vi "Get Graph Bounds.vi"(0 "eye scan point iterator":refnum<class "niHighSpeedSerial Rectangular Eye Scan Point Iterator v1 Host.lvclass">, 11 "error in":errorcluster) -> (4 "eye scan point iterator out":refnum<class "niHighSpeedSerial Rectangular Eye Scan Point Iterator v1 Host.lvclass">, 6 "x scale.range":T2, 8 "x scale.offset and multiplier":T1, 10 "y scale.range":T2, 14 "y scale.offset and multiplier":T1, 15 "error out":errorcluster)   [LabVIEW 2014, in "niHighSpeedSerial Rectangular Eye Scan Point Iterator v1 Host.lvclass"]
doc: "Returns the x, y, and z bounds to format an Intensity Graph based on the configuration of the Eye Scan Point Iterator object.\n\n<B>Input Parameters</B>\n\n<B>eye scan point iterator</B> is the incoming wire for the Eye Scan Point Iterator class object.\n\n<B>error in</B> describes error conditions that occur before this node runs. This input provides standard 'error in' functionality.\n\n<B>Output Parameters</B>\n\n<B>eye scan point iterator out</B> is the outgoing wire for the Eye Scan Point Iterator class object.\n\n<B>x scale.range</B> is the range for the x scale.\n\n<B>x scale.range.Minimum</B> is the minimum value for the x scale's range.\n\n<B>x scale.range.Maximum</B> is the maximum value for the x scale's range.\n\n<B>x scale.range.Increment</B> is the increment for the x scale's range.\n\n<B>x scale.range.Minor Increment</B> is the minor increment value for the x scale's range.\n\n<B>x scale.range.Start</B> is the start value for the x scale's range\n\n<B>x scale.offset and multiplier</B> is the offset and multiplier for the x scale's range.\n\n<B>x scale.offset and multiplier.Offset</B> is the offset for the x scale's range.\n\n<B>x scale.offset and multiplier.Multiplier</B> is the multiplier for the x scale's range.\n\n<B>y scale.range</B> is the range for the y scale.\n\n<B>y scale.range.Minimum</B> is the minimum value for the y scale's range.\n\n<B>y scale.range.Maximum</B> is the maximum value for the y scale's range.\n\n<B>y scale.range.Increment</B> is the increment for the y scale's range.\n\n<B>y scale.range.Minor Increment</B> is the minor increment for the y scale's range.\n\n<B>y scale.range.Start</B> is the start value for the y scale's range.\n\n<B>y scale.offset and multiplier</B> is the offset and multiplier for the y scale's range.\n\n<B>y scale.offset and multiplier.Offset</B> is the offset for the y scale's range.\n\n<B>y scale.offset and multiplier.Multiplier</B> is the multiplier for the y scale's range.\n\n<B>error out</B> contains error information. This output provides standard 'error out' functionality."
uses:
  <instrlib>/niHighSpeedSerial/Eye Scan/v1/Host/Impl/Rect Iter/niHighSpeedSerial Rectangular Eye Scan Point Iterator v1 Host.lvclass
  <vilib>/Utility/miscctls.llb/LVRangeTypeDef.ctl
  <vilib>/Utility/miscctls.llb/LVOffsetAndMultiplierTypeDef.ctl
  <instrlib>/niHighSpeedSerial/Eye Scan/v1/Host/Impl/Rect Iter/niHighSpeedSerial Rectangular Eye Scan Point Iterator v1 Host.lvclass/niHighSpeedSerial Rectangular Eye Scan Point Iterator v1 Host.ctl
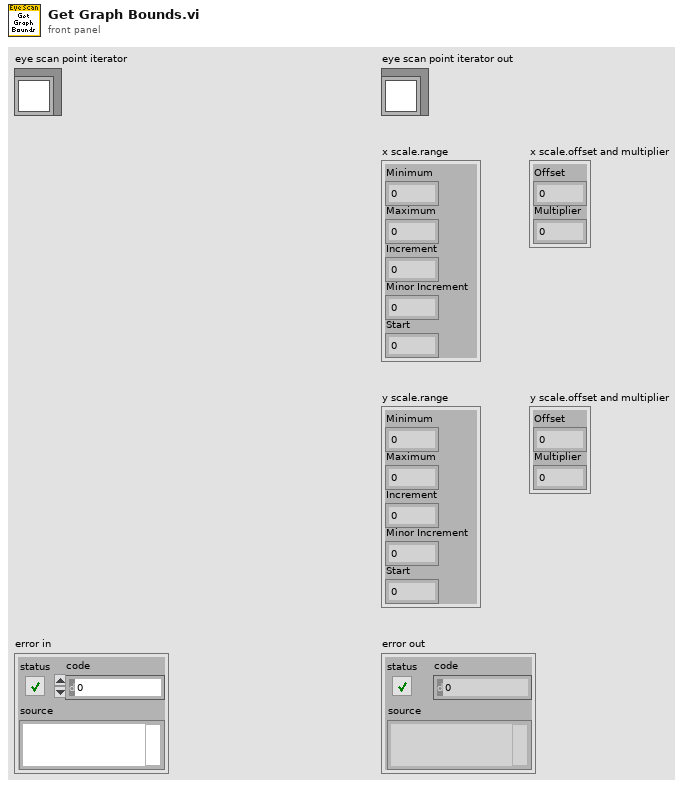
[diagram p1: front panel]
types:
  T1 = typedef "LVOffsetAndMultiplierTypeDef.ctl" = cluster{"Offset":dbl, "Multiplier":dbl}
  T2 = typedef "LVRangeTypeDef.ctl" = cluster{"Minimum":dbl, "Maximum":dbl, "Increment":dbl, "Minor Increment":dbl, "Start":dbl}
  T3 = typedef "niHighSpeedSerial Eye Scan Common v1 Host.lvlib/Point.ctl" = cluster{"point offsets":T4, "sample count":u64, "error count":u64, "bit error rate":dbl}
  T4 = typedef "niHighSpeedSerial Eye Scan Common v1 Host.lvlib/Point Offsets.ctl" = cluster{"horizontal offset":i16, "vertical offset":i8}
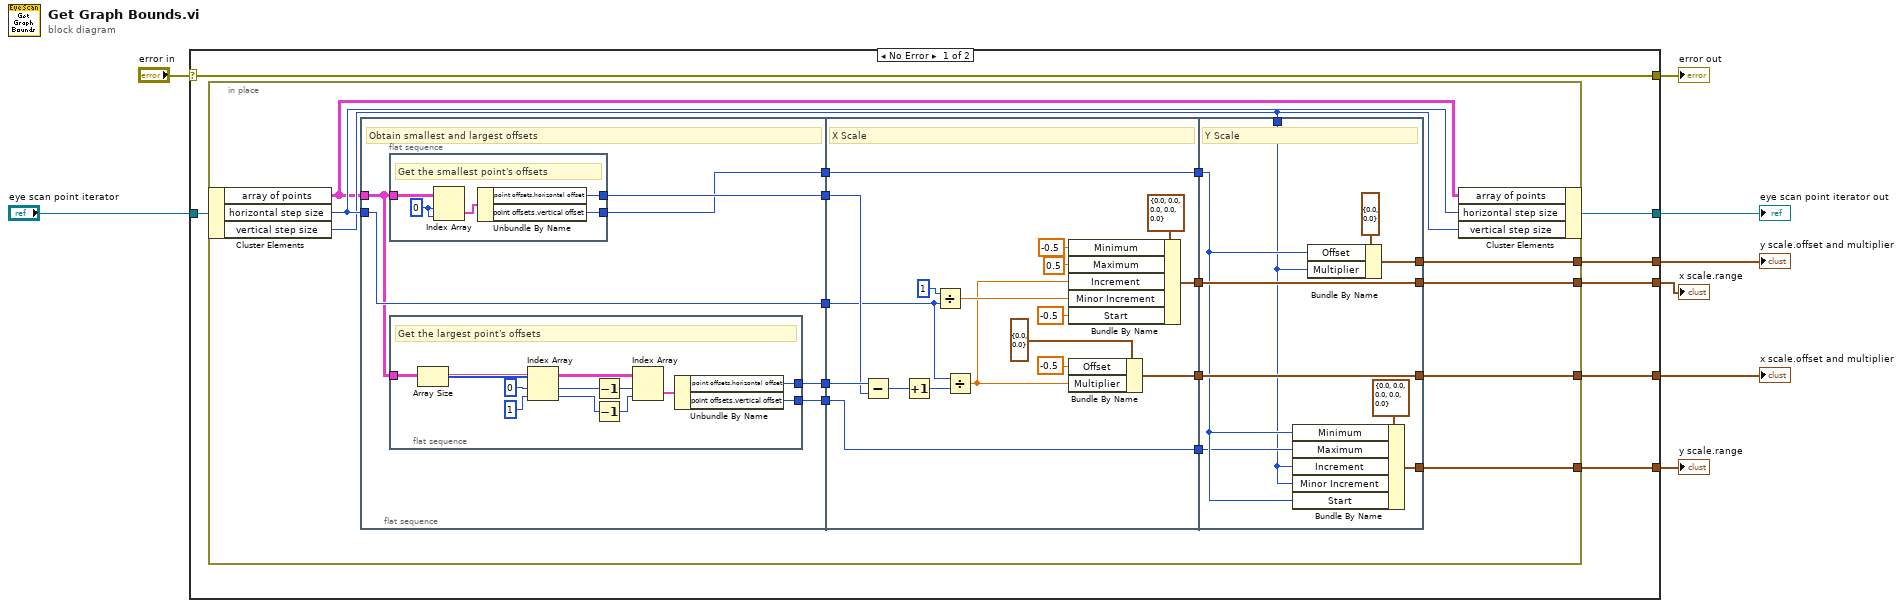
[diagram p0: block diagram]
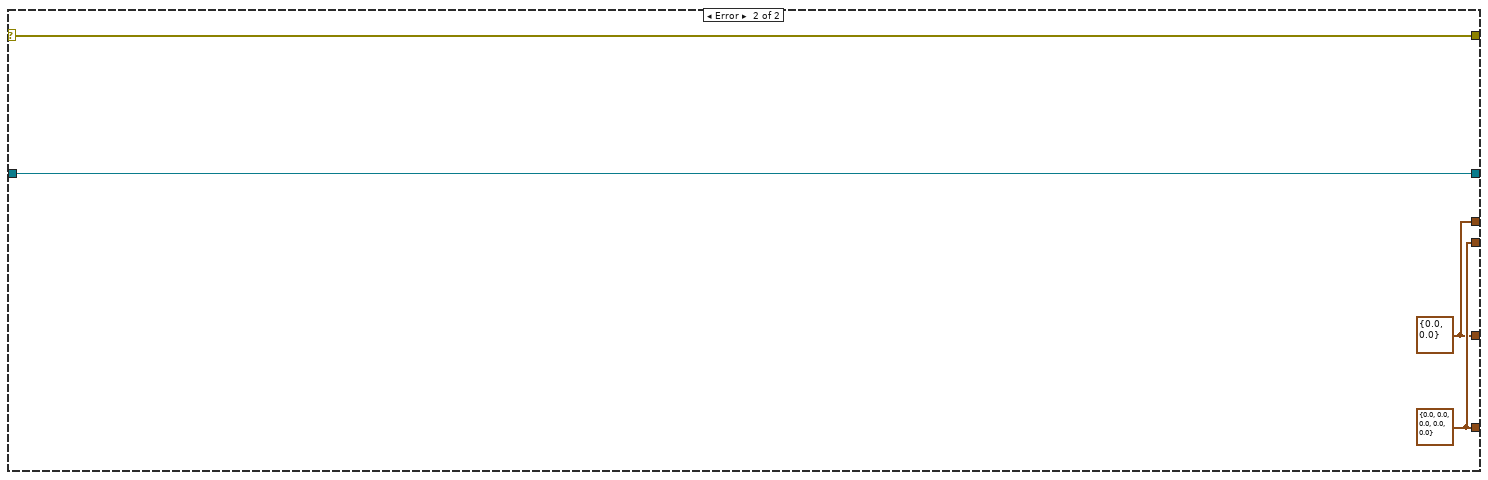
[diagram p2: hidden frame]
diagram:
  n1 = case shown="No Error" "error in" {
    selector: "error in" -> [w15 w84]
    tunnel: [w15 w84] -> w7
    tunnel: [w9 w83] -> w6
    tunnel: "eye scan point iterator" -> [w10 w83]
    tunnel: [w13 w82] -> w4
    tunnel: [w11 w81] -> w3
    tunnel: [w14 w82] -> w2
    tunnel: [w12 w81] -> w1
    frame No Error {
      n2 = in-place {
        in-place-border: [w29] -> w14
        in-place-border: [w26] -> w13
        in-place-border: [w30] -> w12
        in-place-border: [w24] -> w11
        n3 = in-place-cluster #1(w10) -> ("array of points"=w20:T3[][], "horizontal step size"=w31:i16, "vertical step size"=w25:i16)
        n4 = flat-sequence {
          tunnel: w31 -> [w37]
          tunnel: [w37] -> w23
          tunnel: [w34] -> w22
          tunnel: [w36] -> w21
          tunnel: w20 -> [w33]
          tunnel: [w35] -> w18
          tunnel: [w32] -> w16
          tunnel: [w65] -> w28
          tunnel: [w58] -> w27
          tunnel: w23 -> [w60]
          tunnel: w22 -> [w67]
          tunnel: w21 -> [w66]
          tunnel: [w56] -> w19
          tunnel: w18 -> [w56]
          tunnel: [w55] -> w17
          tunnel: w16 -> [w55]
          tunnel: [w79] -> w29
          tunnel: [w80] -> w30
          tunnel: w28 -> [w80]
          tunnel: w27 -> [w79]
          tunnel: [w77] -> w26
          tunnel: w25 -> [w72]
          tunnel: [w75] -> w24
          tunnel: w19 -> [w74]
          tunnel: w17 -> [w73]
          frame #0 {
            # "Obtain smallest and largest offsets"
            n5 = flat-sequence {
              tunnel: [w51] -> w35
              tunnel: w33 -> [w50]
              tunnel: [w49] -> w36
              frame #0 {
                w53 = 0 ("index (row)")
                # "Get the smallest point's offsets"
                n6 = Index Array(array=w50, index (row)=w53, index (col)=w53) -> (element=w52:T3)
                n7 = Unbundle By Name(w52) -> ("point offsets.horizontal offset"=w49:i16, "point offsets.vertical offset"=w51:i8)
              }
            }
            n8 = flat-sequence {
              tunnel: w33 -> [w45]
              tunnel: [w41] -> w32
              tunnel: [w38] -> w34
              frame #0 {
                # "Get the largest point's offsets"
                n9 = Array Size(array=w45) -> (size(s)=w48:i32[])
                n10 = Index Array(array=w48, index #1=0 ("index"), index #2=1 ("index")) -> (element #1=w44:i32, element #2=w43:i32)
                n11 = Decrement(x=w44) -> (x-1=w40:i32)
                n12 = Decrement(x=w43) -> (x-1=w39:i32)
                n13 = Index Array(array=w45, index (row)=w40, index (col)=w39) -> (element=w42:T3)
                n14 = Unbundle By Name(w42) -> ("point offsets.horizontal offset"=w38:i16, "point offsets.vertical offset"=w41:i8)
              }
            }
          }
          frame #1 {
            # "X Scale"
            n15 = Subtract(x=w67, y=w66) -> (x-y=w70:i16)
            n16 = Increment(x=w70) -> (x+1=w71:i16)
            n17 = Divide(x=i16 1, y=w60) -> (x/y=w64:dbl)
            n18 = Divide(x=w60, y=w71) -> (x/y=w59:dbl)
            n19 = Bundle By Name ("X Scale.Range")(cluster=T2 {"Minimum"=0.0, "Maximum"=0.0, "Increment"=0.0, "Minor Increment"=0.0, "Start"=0.0} ("X Scale.Range"), "Minimum"=-0.5 ("Minor Increment"), "Maximum"=0.5, "Increment"=w59, "Minor Increment"=w64, "Start"=-0.5) -> (w58:T2)
            n20 = Bundle By Name ("X Scale.Offset and Multiplier")(cluster=T1 {"Offset"=0.0, "Multiplier"=0.0} ("X Scale.Offset and Multiplier"), "Offset"=-0.5, "Multiplier"=w59) -> (w65:T1)
          }
          frame #2 {
            # "Y Scale"
            n21 = Bundle By Name ("Y Scale.Range")(cluster=T2 {"Minimum"=0.0, "Maximum"=0.0, "Increment"=0.0, "Minor Increment"=0.0, "Start"=0.0} ("input cluster"), "Minimum"=w74, "Maximum"=w73, "Increment"=w72, "Minor Increment"=w72, "Start"=w74) -> (w77:T2)
            n22 = Bundle By Name ("Y Scale.Offset and Multiplier")(cluster=T1 {"Offset"=0.0, "Multiplier"=0.0} ("Y Scale.Offset and Multiplier"), "Offset"=w74, "Multiplier"=w72) -> (w75:T1)
          }
        }
        n23 = in-place-cluster #1("array of points"=w20, "horizontal step size"=w31, "vertical step size"=w25) -> (w9:refnum<class "niHighSpeedSerial Rectangular Eye Scan Point Iterator v1 Host.lvclass">)
      }
    }
    frame Error {
      w81 = T1 {"Offset"=0.0, "Multiplier"=0.0} ("Y Scale.Offset and Multiplier")
      w82 = T2 {"Minimum"=0.0, "Maximum"=0.0, "Increment"=0.0, "Minor Increment"=0.0, "Start"=0.0} ("X Scale.Range")
    }
  }
  "error out" <- w7
  "eye scan point iterator out" <- w6
  "x scale.range" <- w2
  "y scale.range" <- w4
  "x scale.offset and multiplier" <- w1
  "y scale.offset and multiplier" <- w3
